vi "MIDIInEvents.get.vi"(11 "midi-callback-userevent":refnum<class "midi-callback-userevent.lvclass">) -> (2 "MIDIInEvents":refnum<user-event>)   [LabVIEW 2020, in "midi-callback-userevent.lvclass"]
uses:
  midi-callback-userevent.lvclass
  midi-callback-userevent.lvclass/midi-callback-userevent.ctl
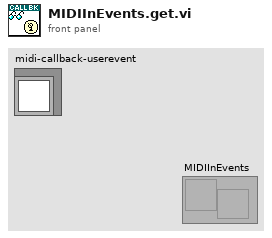
[diagram p1: front panel]
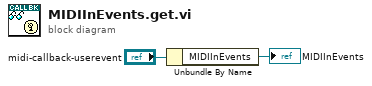
[diagram p0: block diagram]
diagram:
  n1 = Unbundle By Name("midi-callback-userevent") -> ("MIDIInEvents"=→"MIDIInEvents":refnum<user-event>)
